vi "ReceivePass.vi"(8 "error in (no error)":errorcluster, 9 "Ball":refnum<class "Ball.lvclass">, 10 "Robot in":refnum<class "Robot.lvclass">, 11 "AlignSkill in":refnum<class "AlignSkill.lvclass">) -> (0 "error out":errorcluster, 2 "Robot out":refnum<class "Robot.lvclass">, 3 "AlignSkill out":refnum<class "AlignSkill.lvclass">)   [LabVIEW 2023, in "AlignSkill.lvclass"]
uses:
  AlignSkill.lvclass
  Ball_class/Ball.lvclass
  C:/Users/ebert/Documents/codes/SSL/repo/SSL_AI/Object_class/Object.lvclass
  Robot_class/Robot.lvclass
  Object_class/Object.lvclass/Object.ctl
  Ball_class/Ball.lvclass/Ball.ctl
  <vilib>/Analysis/baseanly.llb/Unit Vector (DBL).vi
  Object_class/Read position(x,y).vi
  Ball_class/Read v_x.vi
  Ball_class/Read v_y.vi
  Ball_class/Read velocityNorm.vi
  <vilib>/Analysis/_algsub.llb/Vector Norm.vi
  <vilib>/Analysis/_algsub.llb/Real Vector Norm.vi
  <vilib>/Analysis/NI_AALBase.lvlib
  Utilities_class/Utilities.lvclass
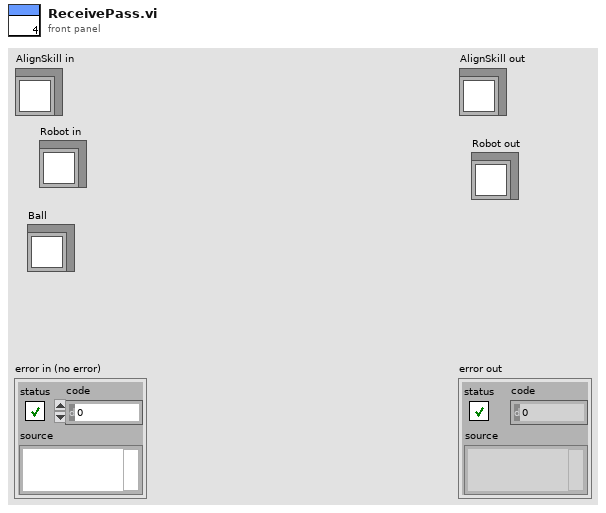
[diagram p1: front panel]
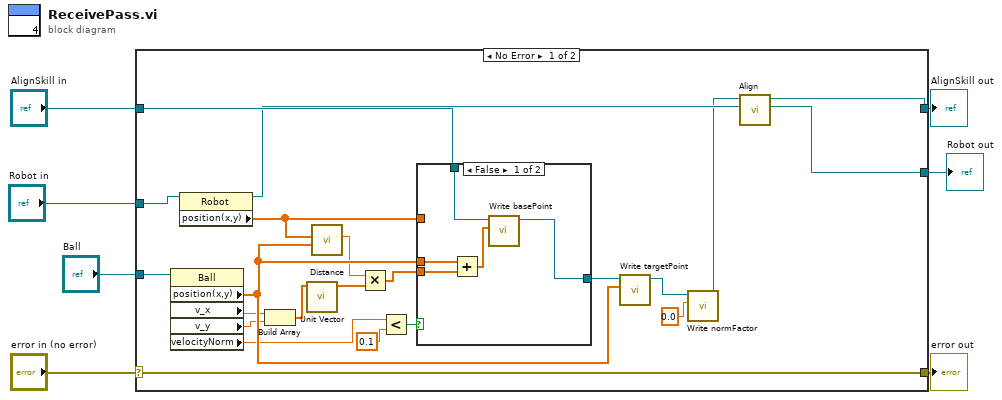
[diagram p0: block diagram]
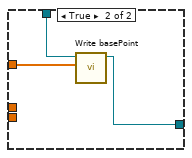
[diagram p2: hidden frame]
diagram:
  n1 = case shown="No Error" "error in (no error)" {
    selector: "error in (no error)" -> [w29 w40]
    tunnel: [w29 w40] -> w6
    tunnel: [w23 w39] -> w4
    tunnel: "AlignSkill in" -> [w25 w39]
    tunnel: "Ball" -> [w28 _]
    tunnel: "Robot in" -> [w24 w38]
    tunnel: [w22 w38] -> w1
    frame No Error {
      n2 = property class="Ball"(reference=w28) -> ("position(x,y)"=w18:dbl[], "v_x"=w10:dbl, "v_y"=w11:dbl, "velocityNorm"=w9:dbl)  [unwired: 1 in, 2 out]
      n3 = property class="Robot"(reference=w24) -> (reference out=w21:refnum<class "Robot.lvclass">, "position(x,y)"=w19:dbl[])  [unwired: 1 in, 1 out]
      n4 = Build Array(w10, w11) -> (w20:dbl[])
      n5 = call-poly <vilib>:"Unit Vector.vi"("Input Vector"=w20) -> ("Unit Vector"=w8:dbl[])  [unwired: 8 in, 2 out]
      n6 = call "Distance.vi"("P1"=w18, "P2"=w19) -> ("Distance"=w17:dbl)  [unwired: 7 in, 2 out]
      n7 = Multiply(x=w17, y=w8) -> (x*y=w16:dbl[])
      n8 = Less?(x=w9, y=0.1) -> (x < y?=w26:bool)
      n9 = case shown="False" w26 {
        tunnel: w25 -> [w32 w37]
        tunnel: w19 -> [_ w36]
        tunnel: w18 -> [w34 _]
        tunnel: w16 -> [w33 _]
        tunnel: [w30 w35] -> w13
        frame False {
          n10 = Add(x=w34, y=w33) -> (x+y=w31:dbl[])
          n11 = call-dynamic "Write basePoint.vi"("basePoint"=w31, "AlignSkill in"=w32) -> ("AlignSkill out"=w30:refnum<class "AlignSkill.lvclass">)  [unwired: 8 in, 1 out]
        }
        frame True {
          n12 = call-dynamic "Write basePoint.vi"("basePoint"=w36, "AlignSkill in"=w37) -> ("AlignSkill out"=w35:refnum<class "AlignSkill.lvclass">)  [unwired: 8 in, 1 out]
        }
      }
      n13 = call-dynamic "Write targetPoint.vi"("targetPoint"=w18, "AlignSkill in"=w13) -> ("AlignSkill out"=w15:refnum<class "AlignSkill.lvclass">)  [unwired: 8 in, 1 out]
      n14 = call-dynamic "Write normFactor.vi"("normFactor"=0.0, "AlignSkill in"=w15) -> ("AlignSkill out"=w12:refnum<class "AlignSkill.lvclass">)  [unwired: 8 in, 1 out]
      n15 = call-dynamic "Align.vi"("Robot"=w21, "AlignSkill in"=w12) -> ("Robot out"=w22:refnum<class "Robot.lvclass">, "AlignSkill out"=w23:refnum<class "AlignSkill.lvclass">)  [unwired: 7 in, 1 out]
    }
    frame Error {
    }
  }
  "error out" <- w6
  "AlignSkill out" <- w4
  "Robot out" <- w1
